vi "nanocal -- nuclear schottky fit V5.vi"() -> ()   [LabVIEW 2020] (continued)
                tunnel: [w595] -> w572 mode=indexing
                tunnel: w557 -> [w594] mode=indexing
                i -> [w596]
                n260 = Number To Fractional String(number=w594, precision (6)=i16 3) -> (F-format string=w595:string)  [unwired: 2 in]
                n261 = Insert Into Map(map in=w598, key=w596, value=w594) -> (map out=w597:map{i32, dbl})  [unwired: 2 out]
              }
              n262 = property on="θ (deg)" class="Ring (strict)"("Strings []"=w571) -> ()  [unwired: 2 in, 2 out]
              n263 = property on="B (T)" class="Ring (strict)"("Strings []"=w572) -> ()  [unwired: 2 in, 2 out]
              n264 = in-place-cluster #4("lookup.all set of"=w561, "lookup.all sides"=w560, "lookup.all T's"=w559, "lookup.all θ's"=w558, "lookup.all B's"=w557, "lookup.set of lookup"=w566, "lookup.side lookup"=w565, "lookup.T lookup"=w563, "lookup.B lookup"=w564, "lookup.θ lookup"=w562) -> (w541:T15)
            }
            n265 = for {
              tunnel: w545 -> [w609] mode=indexing
              shift-right: [w607] -> w543
              shift-left: w544 -> [w608]
              n266 = Unbundle(w609) -> ("event data"=w605:string, "file pattern"=w606:string)
              n267 = Insert Into Map(map in=w608, key=w606, value=w605) -> (map out=w607:map{string, string})  [unwired: 2 out]
            }
            n268 = local read "temps&degs"() -> (w549:map{string, map{T4, dbl}})
            n269 = local read "X selector"() -> (w548:T4)
            n270 = for {
              tunnel: [w618] -> w553 mode=indexing
              tunnel: [w622] -> w551 mode=indexing
              tunnel: [w619] -> w555 mode=indexing
              tunnel: w548 -> [w623]
              tunnel: w543 -> [w621] mode=indexing
              tunnel: w549 -> [w620]
              n271 = Unbundle(w621) -> (w618:string, w619:string)
              n272 = Look In Map(map=w620, key=w619) -> (value=w624:map{T4, dbl})  [unwired: 1 in, 1 out]
              n273 = Look In Map(map=w624, key=w623) -> (value=w622:dbl)  [unwired: 1 in, 1 out]
            }
            n274 = call "array - sorted inexes.vi"("x"=w551) -> ("index array"=w552:i32[])  [unwired: 9 in, 1 out]
            n275 = for {
              tunnel: w552 -> [w614] mode=indexing
              tunnel: w553 -> [w617]
              tunnel: [w616] -> w554 mode=indexing
              tunnel: w555 -> [w615]
              shift-right: [w610] -> w556
              shift-left: w550 -> [w613]
              i -> [w612]
              n276 = Index Array(array=w617, index=w614) -> (element=w616:string)
              n277 = Index Array(array=w615, index=w614) -> (element=w611:string)
              n278 = Insert Into Map(map in=w613, key=w612, value=w611) -> (map out=w610:map{i32, string})  [unwired: 2 out]
            }
            "filesnames lookup" <- w556
            n279 = property on="filenames" class="Ring (strict)"("Strings []"=w554) -> ()  [unwired: 2 in, 2 out]
            n280 = Generate User Event(user event=w546, event data cluster="action: update state of selectors" ("event data")) -> ()  [unwired: 2 in, 2 out]
            n281 = local write "selector"(w541) -> ()
          }
          frame "action: update constrained file selector" {
            w631 = map{i32, string} {}  # Size: 0
            n282 = local read "state of all selectors"() -> (w627:map{T4, map{bool, dbl}})
            n283 = local read "all short filenames"() -> (w628:map{string, string})
            n284 = local read "temps&degs"() -> (w629:map{string, map{T4, dbl}})
            n285 = for {
              tunnel: w628 -> [w641] mode=indexing
              tunnel: [w641] -> w630 mode=indexing if=w637
              shift-right: [w640] -> w626
              shift-left: w629 -> [w640]
              tunnel: w627 -> [w638]
              n286 = for {
                tunnel: [w653] -> w639 mode=indexing
                shift-right: [w648] -> _
                shift-left: w641 -> [w648]
                shift-right: [w647] -> _
                shift-left: w640 -> [w647]
                tunnel: w638 -> [w646] mode=indexing
                n287 = Unbundle(w648) -> ("event data"=w652:string)  [unwired: 1 out]
                n288 = Unbundle(w646) -> ("Plost: sweep window"=w645:T4, "map"=w644:map{bool, dbl})
                n289 = for {
                  tunnel: w644 -> [w656] mode=indexing
                  tunnel: [w655] -> w642
                  tunnel: [w654] -> w643
                  n290 = Unbundle(w656) -> ("ignore side !"=w655:bool, "number OUT"=w654:dbl)
                }
                n291 = Look In Map(map=w647, key=w652) -> (value=w651:map{T4, dbl})  [unwired: 1 in, 1 out]
                n292 = Look In Map(map=w651, key=w645) -> (value=w650:dbl)  [unwired: 1 in, 1 out]
                n293 = Equal?(x=w650, y=w643) -> (x = y?=w649:bool)
                n294 = Or(x=w642, y=w649) -> (x .or. y?=w653:bool)
              }
              n295 = And Array Elements(Boolean array=w639) -> (logical AND=w637:bool)
            }
            n296 = for {
              tunnel: [w671] -> w634 mode=indexing
              tunnel: [w669] -> w632 mode=indexing
              tunnel: [w666] -> w636 mode=indexing
              tunnel: w630 -> [w668] mode=indexing
              tunnel: w626 -> [w667]
              n297 = Unbundle(w668) -> ("event data"=w666:string, "file pattern"=w671:string)
              n298 = local read "X selector"() -> (w665:T4)
              n299 = Look In Map(map=w667, key=w666) -> (value=w670:map{T4, dbl})  [unwired: 1 in, 1 out]
              n300 = Look In Map(map=w670, key=w665) -> (value=w669:dbl)  [unwired: 1 in, 1 out]
            }
            n301 = call "array - sorted inexes.vi"("x"=w632) -> ("index array"=w633:i32[])  [unwired: 9 in, 1 out]
            n302 = for {
              tunnel: w633 -> [w661] mode=indexing
              tunnel: w634 -> [w664]
              tunnel: [w663] -> w635 mode=indexing
              tunnel: w636 -> [w662]
              shift-right: [w657] -> w625
              shift-left: w631 -> [w660]
              i -> [w659]
              n303 = Index Array(array=w664, index=w661) -> (element=w663:string)
              n304 = Index Array(array=w662, index=w661) -> (element=w658:string)
              n305 = Insert Into Map(map in=w660, key=w659, value=w658) -> (map out=w657:map{i32, string})  [unwired: 2 out]
            }
            "constrained filename lookup" <- w625
            n306 = property on="selection :|\\" class="Ring (strict)"("Strings []"=w635) -> ()  [unwired: 2 in, 2 out]
          }
          frame "action: constrained filenames select" {
            (unwired) 1
            n307 = local read "constrained filename lookup"() -> (w674:map{i32, string})
            n308 = local read "selection :|\\"() -> (w675:u16)
            n309 = local read "all full filenames"() -> (w676:map{string, path})
            n310 = Look In Map(map=w674, key=w675) -> (value=w677:string)  [unwired: 1 in, 1 out]
            n311 = Look In Map(map=w676, key=w677) -> (value=w678:path)  [unwired: 1 in, 1 out]
            n312 = local write "Read from file"(w678) -> ()
            n313 = Generate User Event(user event=w673, event data cluster="action: read from file" ("event data")) -> ()  [unwired: 2 in, 2 out]
          }
          frame "action: write mathematica string" {
            n314 = local read "mathematica thing"() -> (w683:map{string, map{T4, dbl}})
            n315 = local read "folder"() -> (w682:path)
            n316 = Build Path(base path=w682, name or relative path="temporarystring.txt") -> (appended path=w681:path)
            n317 = call "string parse mathematica list assosiated array -- V2.vi"("action"=3-lorentzian-heat-response_action."create string" ("derivative"), "Map IN"=w683) -> ("string out"=w679:string)  [unwired: 8 in, 1 out]
            "string OUT" <- w679
            n318 = Write to Text File(file (use dialog)=w681, text=w679) -> ()  [unwired: 2 in, 3 out]
          }
          frame "action: replot colors" {
            # "all -- including kappa0"
            n319 = local read "state of all selectors string"() -> (w692:string)
            n320 = local read "new selector names"() -> (w697:map{T4, map{T13, string}})
            n321 = local read "X selector"() -> (w693:T4)
            n322 = Look In Map(map=w697, key=w693) -> (value=w696:map{T13, string})  [unwired: 1 in, 1 out]
            n323 = local read "state of all selectors"() -> (w704:map{T4, map{bool, dbl}})
            n324 = local read "mathematica thing"() -> (w705:map{string, map{T4, dbl}})
            n325 = Look In Map(map=w696, key=nameformattingitem."nameL") -> (value=w694:string)  [unwired: 1 in, 1 out]
            n326 = Concatenate Strings(w692, w694) -> (w703:string)
            n327 = for {
              tunnel: w705 -> [w726]
              tunnel: w693 -> [w721]
              tunnel: w687 -> [w709] mode=indexing
              tunnel: w704 -> [w722]
              tunnel: w697 -> [w713]
              shift-right: [w717] -> w691
              shift-left: w703 -> [w720]
              tunnel: w692 -> [w718]
              tunnel: [w714] -> w690 mode=indexing
              n328 = for {
                tunnel: w726 -> [w740] mode=indexing
                tunnel: w709 -> [w739]
                tunnel: [w738] -> w725 mode=indexing if=w732
                tunnel: [w737] -> w724 mode=indexing if=w732
                tunnel: w721 -> [w736]
                tunnel: w722 -> [w735]
                n329 = Unbundle(w740) -> ("Map"=w734:map{T4, dbl})  [unwired: 1 out]
                n330 = for {
                  tunnel: w735 -> [w749] mode=indexing
                  tunnel: w734 -> [w748]
                  tunnel: [w746] -> w733 mode=indexing
                  n331 = Unbundle(w749) -> ("Plost: sweep window"=w747:T4, "map"=w745:map{bool, dbl})
                  n332 = for {
                    tunnel: w745 -> [w752] mode=indexing
                    tunnel: [w751] -> w742
                    tunnel: [w750] -> w743
                    n333 = Unbundle(w752) -> ("ignore side !"=w751:bool, "number OUT"=w750:dbl)
                  }
                  n334 = Look In Map(map=w748, key=w747) -> (value=w744:dbl)  [unwired: 1 in, 1 out]
                  n335 = Equal?(x=w744, y=w743) -> (x = y?=w741:bool)
                  n336 = Or(x=w742, y=w741) -> (x .or. y?=w746:bool)
                }
                n337 = Look In Map(map=w734, key=w736) -> (value=w738:dbl)  [unwired: 1 in, 1 out]
                n338 = Look In Map(map=w734, key=w739) -> (value=w737:dbl)  [unwired: 1 in, 1 out]
                n339 = And Array Elements(Boolean array=w733) -> (logical AND=w732:bool)
              }
              n340 = Look In Map(map=w713, key=w709) -> (value=w711:map{T13, string})  [unwired: 1 in, 1 out]
              n341 = Look In Map(map=w711, key=nameformattingitem."nameL") -> (value=w710:string)  [unwired: 1 in, 1 out]
              n342 = call <vilib>:"Space Constant.vi"() -> ("String"=w719:string)
              n343 = Concatenate Strings(w720, w719, w718, w710) -> (w717:string)
              n344 = call "array - sorted inexes.vi"("x"=w725) -> ("index array"=w723:i32[])  [unwired: 9 in, 1 out]
              n345 = for {
                tunnel: w725 -> [w731]
                tunnel: w724 -> [w730]
                tunnel: w723 -> [w727] mode=indexing
                tunnel: [w729] -> w716 mode=indexing
                tunnel: [w728] -> w715 mode=indexing
                n346 = Index Array(array=w731, index=w727) -> (element=w729:dbl)
                n347 = Index Array(array=w730, index=w727) -> (element=w728:dbl)
              }
              n348 = Bundle(w716, w715) -> (w714:cluster{dbl[], dbl[]})  [unwired: 1 in]
            }
            n349 = local read "folder"() -> (w702:path)
            n350 = Concatenate Strings("plotstring", w692, ".dat") -> (w698:string)
            n351 = Build Path(base path=w702, name or relative path=w698) -> (appended path=w701:path)
            n352 = call "nanocal -- plotstring file manage.vi"("Enum"=nanocal_--_plotstring_file_action."generate plotstring thing", "all data"=w690, "header line"=w691) -> ("plotstring thing"=w688:string)  [unwired: 8 in]
            n353 = flat-sequence {
              tunnel: w690 -> [w706]
              tunnel: w686 -> [w708]
              tunnel: "interface: replot colors plot" ("event data") -> [w707]
              frame #0 {
                "color data" <- w706
              }
              frame #1 {
                n354 = Generate User Event(user event=w708, event data cluster=w707) -> ()  [unwired: 2 in, 2 out]
              }
            }
            n355 = Write to Text File(file (use dialog)=w701, text=w688) -> ()  [unwired: 2 in, 3 out]
          }
          frame "action: update state of selectors" {
            w773 = T4[] [enum."T (K)", enum."B (T)", enum."θ (deg)", enum."side (S|R)"] items=["ζ", "τ1", "τS", "τN", "τC", "κ0", "m1", "m2", "m3", "T (K)", "B (T)", "θ (deg)", "side (S|R)", "set of (B|T)", "Re(offset)", "Im(offset)"]
            n356 = local read "selector"() -> (w769:T15)
            n357 = Unbundle By Name(w769) -> ("side (8S|4R)"=w768:i32, "ignore side !"=w767:bool, "lookup.side lookup"=w766:map{i32, dbl}, "T (K)"=w763:u16, "ignore T !"=w765:bool, "lookup.T lookup"=w764:map{i32, dbl}, "B (T)"=w760:u16, "ignore B !"=w762:bool, "lookup.B lookup"=w761:map{i32, dbl}, "θ (deg)"=w758:u16, "ignore θ !"=w757:bool, "lookup.θ lookup"=w759:map{i32, dbl}, "set (1T|2B)"=w754:i32, "ignore set of !"=w755:bool, "lookup.set of lookup"=w756:map{i32, dbl})
            n358 = Look In Map(map=w766, key=w768) -> (value=w772:dbl)  [unwired: 1 in, 1 out]
            n359 = local read "new selector names"() -> (w776:map{T4, map{T13, string}})
            n360 = node(w767, w772) -> (w793:map{bool, dbl})
            n361 = Look In Map(map=w764, key=w763) -> (value=w792:dbl)  [unwired: 1 in, 1 out]
            n362 = Look In Map(map=w761, key=w760) -> (value=w788:dbl)  [unwired: 1 in, 1 out]
            n363 = node(w765, w792) -> (w790:map{bool, dbl})
            n364 = node(w762, w788) -> (w787:map{bool, dbl})
            n365 = Look In Map(map=w759, key=w758) -> (value=w786:dbl)  [unwired: 1 in, 1 out]
            n366 = node(w757, w786) -> (w784:map{bool, dbl})
            n367 = Look In Map(map=w756, key=w754) -> (value=w783:dbl)  [unwired: 1 in, 1 out]
            n368 = local read "side map from NUM"() -> (w770:map{i32, T11})
            n369 = node(w755, w783) -> (w781:map{bool, dbl})
            n370 = node(3-lorentzian-parameters."side (S|R)" ("Plost: sweep window"), w793, 3-lorentzian-parameters."T (K)" ("Plost: sweep window"), w790, 3-lorentzian-parameters."B (T)" ("Plost: sweep window"), w787, 3-lorentzian-parameters."θ (deg)" ("Plost: sweep window"), w784, 3-lorentzian-parameters."set of (B|T)" ("Plost: sweep window"), w781) -> (w753:map{T4, map{bool, dbl}})
            "state of all selectors" <- w753
            n371 = for {
              tunnel: w776 -> [w798]
              shift-right: [w801] -> w774
              shift-left: "_" ("event data") -> [w800]
              tunnel: w773 -> [w797] mode=indexing
              tunnel: w753 -> [w795]
              n372 = Look In Map(map=w795, key=w797) -> (value=w803:map{bool, dbl})  [unwired: 1 in, 1 out]
              n373 = Look In Map(map=w798, key=w797) -> (value=w796:map{T13, string})  [unwired: 1 in, 1 out]
              n374 = for {
                tunnel: w803 -> [w818] mode=indexing
                tunnel: [w817] -> w802
                tunnel: [w816] -> w799
                n375 = Unbundle(w818) -> ("ignore side !"=w817:bool, "number OUT"=w816:dbl)
              }
              n376 = case shown="False" w802 {
                tunnel: [w814 w815] -> w801
                tunnel: w800 -> [w813 w815]
                tunnel: w799 -> [w810 _]
                tunnel: w796 -> [w806 _]
                frame False {
                  n377 = Look In Map(map=w806, key=nameformattingitem."units") -> (value=w807:string)  [unwired: 1 in, 1 out]
                  n378 = Look In Map(map=w806, key=nameformattingitem."prec") -> (value=w804:string)  [unwired: 1 in, 1 out]
                  n379 = Format Value(format string=w804, value (0)=w810) -> (output string=w809:string)  [unwired: 1 in]
                  n380 = Concatenate Strings(w813, "_" ("event data"), w809, w807, "_" ("event data")) -> (w814:string)
                }
                frame True {
                }
              }
            }
            "state of all selectors string" <- w774
            n381 = Look In Map(map=w770, key=w772) -> (value=w771:T11)  [unwired: 1 in, 1 out]
            n382 = local write "side"(w771) -> ()
            n383 = Generate User Event(user event=w777, event data cluster="action: replot colors" ("event data")) -> (user event out=w778:refnum<user-event>)  [unwired: 2 in, 1 out]
            n384 = Generate User Event(user event=w778, event data cluster="action: update constrained file selector" ("event data")) -> ()  [unwired: 2 in, 2 out]
          }
          frame "action: copy from math" {
            w828 = map{T4, bool} {}  # Size: 0
            n385 = local read "default selector"() -> (w827:T14)
            n386 = local read "mathematica thing"() -> (w833:map{string, map{T4, dbl}})
            n387 = case shown="True" "overwrite offset" {
              tunnel: w825 -> [w836 w840]
              tunnel: [w836 w839] -> w824
              frame False {
              }
              frame True {
                n388 = Build Array (concatenate)(w840, 3-lorentzian-parameters."Re(offset)" ("Plost: sweep window"), 3-lorentzian-parameters."Im(offset)" ("Plost: sweep window")) -> (w839:T4[])
              }
            }
            n389 = for {
              shift-right: [w844] -> w826
              shift-left: w828 -> [w845]
              tunnel: w827 -> [w843] mode=indexing
              n390 = Unbundle(w843) -> ("Plost: sweep window"=w842:T4, "used default"=w841:bool)
              n391 = Insert Into Map(map in=w845, key=w842, value=w841) -> (map out=w844:map{T4, bool})  [unwired: 2 out]
            }
            n392 = local read "key"() -> (w832:string)
            n393 = local read "parameter map"() -> (w821:map{T4, dbl})
            n394 = Look In Map(map=w833, key=w832) -> (key not found?=w830:bool, value=w831:map{T4, dbl})  [unwired: 1 in]
            n395 = case shown="False" w830 {
              tunnel: w831 -> [w859 _]
              tunnel: w826 -> [w857 _]
              tunnel: w824 -> [w858 _]
              tunnel: "overwrite offset" -> [w851 w894]
              tunnel: [w850 w894] -> w822
              tunnel: w821 -> [w849 _]
              tunnel: w819 -> [w847 _]
              frame False {
                # "the order of numbers \nMUST corrspond to order\nin the \"parameter\" array"
                n396 = for {
                  tunnel: [w869] -> w856 mode=indexing
                  tunnel: w859 -> [w877]
                  tunnel: w858 -> [w870] mode=indexing
                  tunnel: w857 -> [w876]
                  shift-right: [w871] -> w848
                  shift-left: w849 -> [w872]
                  n397 = Look In Map(map=w876, key=w870, default value=FALSE) -> (value=w875:bool)  [unwired: 1 out]
                  n398 = Look In Map(map=w877, key=w870) -> (value=w874:dbl)  [unwired: 1 in, 1 out]
                  n399 = case shown="True" w875 {
                    tunnel: w874 -> [w880 _]
                    tunnel: w870 -> [_ w881]
                    tunnel: [w880 w882] -> w869
                    frame False {
                    }
                    frame True {
                      n400 = local read "T (K)"() -> (w893:dbl)
                      n401 = local read "B (T)"() -> (w889:dbl)
                      n402 = Divide(x=w889, y=12.0) -> (x/y=w887:dbl)
                      n403 = Equal?(x=3-lorentzian-parameters."τN", y=w881) -> (x = y?=w890:bool)
                      n404 = Square(x=w887) -> (x^2=w886:dbl)
                      n405 = call "nanocal -- defaut parameter manager -- V1.vi"("action"=nanocal_--_defaut_parameter_manager_action--_V1."get logarithmic interp", "T"=w893, "what"=w881) -> ("number"=w884:dbl)  [unwired: 8 in]
                      n406 = Select(t=w886, s=w890, f=1.0) -> (s? t:f=w883:dbl)
                      n407 = Multiply(x=w884, y=w883) -> (x*y=w882:dbl)
                    }
                  }
                  n408 = in-place {
                    in-place-border: w869 -> [w879]
                    in-place-border: LVMapReplaceAction."Modify Entry only if found" ("action") -> [w878]
                    n409 = in-place-map #5(w872, w870) -> ()  [unwired: 1 in, 2 out]
                    n410 = in-place-map #5(w879, w878) -> (w871:map{T4, dbl})  [unwired: 2 out]
                  }
                }
                n411 = flat-sequence {
                  tunnel: w848 -> [w860]
                  tunnel: w847 -> [w862]
                  tunnel: "interface: update list from parameter map" ("event data") -> [w861]
                  frame #0 {
                    n412 = local write "parameter map"(w860) -> ()
                  }
                  frame #1 {
                    n413 = Generate User Event(user event=w862, event data cluster=w861) -> ()  [unwired: 2 in, 2 out]
                  }
                }
                n414 = Index Array(array=w856, index #1=6 ("index"), index #2=7 ("index")) -> (element #1=w853:dbl, element #2=w852:dbl)
                n415 = case shown="True" w851 {
                  selector: w851 -> [w863 w864]
                  tunnel: w853 -> [_ w866]
                  tunnel: w852 -> [_ w865]
                  tunnel: [w863 w864] -> w850
                  frame False {
                  }
                  frame True {
                    n416 = Bundle("number"=w866, "number"=w865) -> (w867:cluster{"number":dbl, "number":dbl})  [unwired: 1 in]
                    n417 = local write "offset Re\noffset Im"(w867) -> ()
                  }
                }
              }
              frame True {
              }
            }
            n418 = case shown="True" w822 {
              tunnel: ["action: new sweep" ("event data") "action: read from file" ("event data")] -> w820
              frame False {
              }
              frame True {
              }
            }
            n419 = Generate User Event(user event=w829, event data cluster=w820) -> ()  [unwired: 2 in, 2 out]
          }
          frame "action: copy to math" {
            w902 = T4[] [enum."T (K)", enum."B (T)", enum."θ (deg)", enum."Re(offset)", enum."Im(offset)"] items=["ζ", "τ1", "τS", "τN", "τC", "κ0", "m1", "m2", "m3", "T (K)", "B (T)", "θ (deg)", "side (S|R)", "set of (B|T)", "Re(offset)", "Im(offset)"]
            n420 = local read "offset Re\noffset Im"() -> (w898:cluster{"Numeric":dbl, "Numeric":dbl})
            n421 = local read "parameter map"() -> (w895:map{T4, dbl})
            n422 = local read "θ (deg)"() -> (w904:dbl)
            n423 = local read "T (K)"() -> (w906:dbl)
            n424 = local read "B (T)"() -> (w905:dbl)
            n425 = Unbundle(w898) -> ("Numeric"=w897:dbl, "Numeric"=w896:dbl)
            n426 = Build Array(w906, w905, w904, w897, w896) -> (w903:dbl[])
            n427 = for {
              tunnel: w903 -> [w912] mode=indexing
              tunnel: w902 -> [w913] mode=indexing
              shift-right: [w914] -> w901
              shift-left: w895 -> [w915]
              n428 = Insert Into Map(map in=w915, key=w913, value=w912) -> (map out=w914:map{T4, dbl})  [unwired: 2 out]
            }
            n429 = local read "mathematica thing"() -> (w909:map{string, map{T4, dbl}})
            n430 = local read "key"() -> (w908:string)
            n431 = call "3-lorentzian-heat-response -- V4.vi"("action"=3-lorentzian-heat-response_action."calc m1m2m3", "Map IN"=w901) -> ("Map OUT"=w900:map{T4, dbl})  [unwired: 7 in, 2 out]
            n432 = in-place {
              in-place-border: w900 -> [w916]
              n433 = in-place-map #6(w909, w908) -> (w919:map{T4, dbl})  [unwired: 1 in, 1 out]
              n434 = for {
                tunnel: w916 -> [w921] mode=indexing
                shift-right: [w924] -> w918
                shift-left: w919 -> [w925]
                shift-right: [w923] -> _
                shift-left: w916 -> [w923]
                n435 = Unbundle(w921) -> ("X selector"=w920:T4)  [unwired: 1 out]
                n436 = Look In Map(map=w923, key=w920) -> (value=w922:dbl)  [unwired: 1 in, 1 out]
                n437 = Insert Into Map(map in=w925, key=w920, value=w922) -> (map out=w924:map{T4, dbl})  [unwired: 2 out]
              }
              n438 = in-place-map #6(w918, LVMapReplaceAction."Modify Entry only if found" ("action")) -> (w907:map{string, map{T4, dbl}})  [unwired: 2 out]
            }
            n439 = local write "mathematica thing"(w907) -> ()
            n440 = Generate User Event(user event=w910, event data cluster="action: replot colors" ("event data")) -> ()  [unwired: 2 in, 2 out]
          }
          frame "action: exit" {
          }
          frame "action: read from file" {
            n441 = local read "Read from file"() -> (w927:path)
            n442 = local read "cursor x selector"() -> (w950:map{T4, dbl})
            n443 = call "file - read-write - list of lines-V2.vi"("read/write control"=file_--_read-write_control."read", "file path"=w927) -> ("header OUT"=w937:string, "list of lines OUT"=w939:string[], "filename out"=w967:string)  [unwired: 7 in]
            n444 = Unbundle("offset Re\noffset Im") -> ("Numeric"=w953:dbl, "Numeric"=w952:dbl)
            n445 = call "filename-manage.vi"("filename-action"=filename-action."get name", "file name IN"=w967) -> ("string OUT"=w936:string)  [unwired: 7 in, 2 out]
            n446 = Re/Im To Complex(1:w952, 2:w953) -> (0:w940:cdb)
            n447 = call "filename-manage.vi"("filename-action"=filename-action."get T", "file name IN"=w936) -> ("number OUT"=w949:dbl, "filename OUT"=w964:string)  [unwired: 7 in, 1 out]
            "T (K)" <- w949
            n448 = case shown="\"raw nanocal\"" "data file formatting" {
              tunnel: [w973 w991 w1027 w1054] -> w961
              tunnel: [w972 w990 w1026 w1053] -> w955
              tunnel: w940 -> [w971 w993 w1022 w1043]
              tunnel: w939 -> [w974 w1001 w1021 w1042]
              tunnel: w937 -> [_ w1002 _ _]
              tunnel: w936 -> [_ w989 _ _]
              tunnel: w927 -> [_ w992 _ _]
              tunnel: "side" -> [_ w988 _ _]
              tunnel: "toggle generate labview files" -> [_ w986 _ _]
              frame "as is", Default {
                n449 = for {
                  tunnel: w974 -> [w985] mode=indexing
                  tunnel: [w980] -> w975 mode=indexing if=w976
                  tunnel: [w979] -> w973 mode=indexing if=w976
                  w981 = 0.0
                  n450 = Scan From String(format string="%f%f%f", input string=w985, initial scan location=u32 0, default 1=w981, default 2=w981, default 3=w981) -> (offset past scan=w977:u32, output 1=w979:dbl, output 2=w983:dbl, output 3=w982:dbl)  [unwired: 1 in, 2 out]
                  n451 = Greater Than 0?(x=w977) -> (x > 0?=w976:bool)
                  n452 = Re/Im To Complex(1:w982, 2:w983) -> (0:w980:cdb)
                }
                n453 = Subtract(x=w975, y=w971) -> (x-y=w972:cdb[])
              }
              frame "raw nanocal" {
                n454 = case shown="\"ref\"" w988 {
                  tunnel: [nanocal_raw_file_manage_action_V1."read S side" ("action") nanocal_raw_file_manage_action_V1."read R side" ("action")] -> w987
                  frame "sam", Default {
                  }
                  frame "ref" {
                  }
                }
                n455 = call "nanocal_raw_file_manage_V1.vi"("action"=w987, "list of lines IN"=w1001, "header IN"=w1002) -> ("z (K/W)  OUT"=w994:cdb[], "f (Hz) OUT"=w995:dbl[])  [unwired: 6 in, 1 out]
                n456 = Subtract(x=w994, y=w993) -> (x-y=w996:cdb[])
                n457 = call "array -- freq-voltage transformations.vi"("freq voltage action"=array_--_freq-voltage_transformations_action."add -ω", "z In"=w996, "ω IN"=w995) -> ("z out"=w999:cdb[], "ω out"=w1000:dbl[])  [unwired: 5 in, 2 out]
                n458 = call "array -- freq-voltage transformations.vi"("freq voltage action"=array_--_freq-voltage_transformations_action."sort ω", "z In"=w999, "ω IN"=w1000) -> ("z out"=w990:cdb[], "ω out"=w991:dbl[])  [unwired: 5 in, 2 out]
                n459 = case shown="True" w986 {
                  tunnel: w992 -> [_ w1014]
                  tunnel: w989 -> [_ w1018]
                  tunnel: w991 -> [_ w1010]
                  tunnel: w990 -> [_ w1009]
                  frame False {
                  }
                  frame True {
                    n460 = call "filename-manage.vi"("filename-action"=filename-action."get basename", "file name IN"=w1018) -> ("string OUT"=w1016:string)  [unwired: 7 in, 2 out]
                    n461 = Strip Path(path=w1014) -> (stripped path=w1013:path)  [unwired: 1 out]
                    n462 = Concatenate Strings(w1016, "_labview_.dat") -> (w1005:string)
                    n463 = call "array -- freq-voltage transformations.vi"("freq voltage action"=array_--_freq-voltage_transformations_action."labview file str", "z In"=w1009, "ω IN"=w1010) -> ("lines out"=w1007:string[], "header OUT"=w1008:string)  [unwired: 5 in, 2 out]
                    n464 = Build Path(base path=w1013, name or relative path=w1005) -> (appended path=w1012:path)
                    n465 = call "file - read-write - list of lines-V2.vi"("read/write control"=file_--_read-write_control."write all", "header IN"=w1008, "list of lines IN"=w1007, "file path"=w1012) -> ()  [unwired: 5 in, 3 out]
                  }
                }
              }
              frame "add - ω" {
                n466 = for {
                  tunnel: w1021 -> [w1039] mode=indexing
                  tunnel: [w1034] -> w1023 mode=indexing if=w1030
                  tunnel: [w1033] -> w1019 mode=indexing if=w1030
                  w1035 = 0.0
                  n467 = Scan From String(format string="%f%f%f", input string=w1039, initial scan location=u32 0, default 1=w1035, default 2=w1035, default 3=w1035) -> (offset past scan=w1031:u32, output 1=w1033:dbl, output 2=w1037:dbl, output 3=w1036:dbl)  [unwired: 1 in, 2 out]
                  n468 = Greater Than 0?(x=w1031) -> (x > 0?=w1030:bool)
                  n469 = Re/Im To Complex(1:w1036, 2:w1037) -> (0:w1034:cdb)
                }
                n470 = Subtract(x=w1023, y=w1022) -> (x-y=w1020:cdb[])
                n471 = call "array -- freq-voltage transformations.vi"("freq voltage action"=array_--_freq-voltage_transformations_action."add -ω", "z In"=w1020, "ω IN"=w1019) -> ("z out"=w1028:cdb[], "ω out"=w1029:dbl[])  [unwired: 5 in, 2 out]
                n472 = call "array -- freq-voltage transformations.vi"("freq voltage action"=array_--_freq-voltage_transformations_action."sort ω", "z In"=w1028, "ω IN"=w1029) -> ("z out"=w1026:cdb[], "ω out"=w1027:dbl[])  [unwired: 5 in, 2 out]
              }
              frame "full rydh" {
                n473 = for {
                  tunnel: w1042 -> [w1066] mode=indexing
                  tunnel: [w1061] -> w1044 mode=indexing if=w1057
                  tunnel: [w1060] -> w1040 mode=indexing if=w1057
                  w1062 = 0.0
                  n474 = Scan From String(format string="%f%f%f", input string=w1066, initial scan location=u32 0, default 1=w1062, default 2=w1062, default 3=w1062) -> (offset past scan=w1058:u32, output 1=w1060:dbl, output 2=w1064:dbl, output 3=w1063:dbl)  [unwired: 1 in, 2 out]
                  n475 = Greater Than 0?(x=w1058) -> (x > 0?=w1057:bool)
                  n476 = Re/Im To Complex(1:w1063, 2:w1064) -> (0:w1061:cdb)
                }
                n477 = Subtract(x=w1044, y=w1043) -> (x-y=w1041:cdb[])
                n478 = call "array -- freq-voltage transformations.vi"("freq voltage action"=array_--_freq-voltage_transformations_action."2 x ω", "z In"=w1041, "ω IN"=w1040) -> ("z out"=w1048:cdb[], "ω out"=w1050:dbl[])  [unwired: 5 in, 2 out]
                n479 = call "array -- freq-voltage transformations.vi"("freq voltage action"=array_--_freq-voltage_transformations_action."R-phase(deg) to Re-Im", "z In"=w1048, "ω IN"=w1050) -> ("z out"=w1047:cdb[], "ω out"=w1049:dbl[])  [unwired: 5 in, 2 out]
                n480 = call "array -- freq-voltage transformations.vi"("freq voltage action"=array_--_freq-voltage_transformations_action."add -ω", "z In"=w1047, "ω IN"=w1049) -> ("z out"=w1055:cdb[], "ω out"=w1056:dbl[])  [unwired: 5 in, 2 out]
                n481 = call "array -- freq-voltage transformations.vi"("freq voltage action"=array_--_freq-voltage_transformations_action."sort ω", "z In"=w1055, "ω IN"=w1056) -> ("z out"=w1053:cdb[], "ω out"=w1054:dbl[])  [unwired: 5 in, 2 out]
              }
            }
            n482 = Insert Into Map(map in=w950, key=3-lorentzian-parameters."T (K)" ("Plost: sweep window"), value=w949) -> (map out=w948:map{T4, dbl})  [unwired: 2 out]
            n483 = call "filename-manage.vi"("filename-action"=filename-action."get deg", "file name IN"=w964) -> ("number OUT"=w945:dbl, "filename OUT"=w931:string)  [unwired: 7 in, 1 out]
            "θ (deg)" <- w945
            n484 = local read "side map to STR"() -> (w929:map{T11, string})
            n485 = Insert Into Map(map in=w948, key=3-lorentzian-parameters."θ (deg)" ("Plost: sweep window"), value=w945) -> (map out=w947:map{T4, dbl})  [unwired: 2 out]
            n486 = call "filename-manage.vi"("filename-action"=filename-action."get B", "file name IN"=w931) -> ("number OUT"=w944:dbl, "filename OUT"=w930:string)  [unwired: 7 in, 1 out]
            "B (T)" <- w944
            n487 = call "filename-manage.vi"("filename-action"=filename-action."getIDStock", "file name IN"=w930) -> ("string OUT"=w934:string)  [unwired: 7 in, 2 out]
            "file IDS" <- w934
            n488 = Look In Map(map=w929, key="side") -> (value=w935:string)  [unwired: 1 in, 1 out]
            n489 = Insert Into Map(map in=w947, key=3-lorentzian-parameters."B (T)" ("Plost: sweep window"), value=w944) -> (map out=w946:map{T4, dbl})  [unwired: 2 out]
            n490 = Concatenate Strings(w934, w935) -> (→"key":string)
            n491 = local write "cursor x selector"(w946) -> ()
            n492 = call "filter - complex - four.vi"("omega (Hz) in"=w961, "z in"=w955, "span"="cspan") -> ("omega out"=w960:dbl[], "z out"=w959:cdb[], "dz/domega out"=w958:cdb[])  [unwired: 9 in, 5 out]
            n493 = call "nanocal -- publish -- freq scan V2.vi"("publisher action"=publisher_action."set", "dz/dω IN (V)"=w958, "z IN (V)"=w959, "ω IN (Hz)"=w960) -> ()  [unwired: 4 in, 4 out]
            n494 = Generate User Event(user event=w968, event data cluster="action: new sweep" ("event data")) -> ()  [unwired: 2 in, 2 out]
          }
          frame "action: save freq scan" {
            n495 = local read "Freq sweep name template"() -> (w1072:T10)
            n496 = call "MFLI -- publish -- freq scan.vi"("publisher action"=publisher_action."get") -> ("Voltage out (V)"=w1068:cdb[], "Freq out (Hz)"=w1069:dbl[])  [unwired: 9 in]
            n497 = call "filename-manage.vi"("filename pattern"=w1072, "filename-action"=filename-action."uniquenum", "folder IN"="Save folder", "file name IN"="freq sweep file name") -> ("filename OUT"=w1071:string)  [unwired: 5 in, 2 out]
            n498 = call "KM_appendline -- freq sweep.vi"("freq"=w1069, "Vout(V)"=w1068, "Save frequency scan"="Save folder", "read/write control"=KM_file_--_read-write_control."append one line", "name or relative path"=w1071) -> ()  [unwired: 15 in]
            n499 = local write "freq sweep file name"(w1071) -> ()
          }
          frame "void", Default {
          }
        }
      }
    }
  }
  n500 = while "interface actions" {
    tunnel: w9 -> [w1079]
    tunnel: w6 -> [w1077]
    tunnel: w5 -> [w1076]
    stop <- FALSE stop-if-true
    n501 = event shown="[1] <interface>: User Event" {
      selector: w1079 -> [_ _]
      dyn-events: _ -> [_ _]
      timeout: _ -> [_ _]
      tunnel: w1077 -> [_ w1081]
      tunnel: w1076 -> [_ w1080]
      event Timeout {
        n502 = event-data() -> ()  [unwired: 1 in, 3 out]
      }
      event User Event {
        n503 = event-data() -> ("interface"=w1082:string)  [unwired: 1 in]
        n504 = case shown="\"interface: update curvature plot\"" w1082 {
          tunnel: [_ _ _ _ _ _ _ _ _ _ TRUE] -> _
          tunnel: w1081 -> [_ _ w1103 w1135 _ _ w1204 w1235 _ _ _]
          tunnel: w1080 -> [_ _ _ _ w1153 _ _ _ _ _ _]
          frame "void", Default {
          }
          frame "interface: reset colors" {
            w1089 = map{T4, u32} {}  # Size: 0
            n505 = local read "parameter"() -> (w1092:T4[])
            n506 = local read "colors"() -> (w1090:u32[])
            n507 = for {
              shift-right: [w1101] -> w1091
              shift-left: w1089 -> [w1102]
              tunnel: w1092 -> [w1100] mode=indexing
              tunnel: w1090 -> [w1099] mode=indexing
              n508 = Insert Into Map(map in=w1102, key=w1100, value=w1099) -> (map out=w1101:map{T4, u32})  [unwired: 2 out]
            }
            n509 = local write "color Map"(w1091) -> ()
            n510 = Look In Map(map=w1091, key=3-lorentzian-parameters."ζ" ("Plost: sweep window")) -> (value=w1093:u32)  [unwired: 1 in, 1 out]
            n511 = Look In Map(map=w1091, key=3-lorentzian-parameters."τ1" ("Plost: sweep window")) -> (value=w1094:u32)  [unwired: 1 in, 1 out]
            n512 = Look In Map(map=w1091, key=3-lorentzian-parameters."τS" ("Plost: sweep window")) -> (value=w1095:u32)  [unwired: 1 in, 1 out]
            n513 = Look In Map(map=w1091, key=3-lorentzian-parameters."τN" ("Plost: sweep window")) -> (value=w1096:u32)  [unwired: 1 in, 1 out]
            n514 = Look In Map(map=w1091, key=3-lorentzian-parameters."τC" ("Plost: sweep window")) -> (value=w1097:u32)  [unwired: 1 in, 1 out]
            n515 = Look In Map(map=w1091, key=3-lorentzian-parameters."κ0" ("Plost: sweep window")) -> (value=w1098:u32)  [unwired: 1 in, 1 out]
            n516 = property on="ζ" class="Slide (strict)"("Fill Color"=w1093) -> ()  [unwired: 2 in, 2 out]
            n517 = property on="T1" class="Slide (strict)"("Fill Color"=w1094) -> ()  [unwired: 2 in, 2 out]
            n518 = property on="τS" class="Slide (strict)"("Fill Color"=w1095) -> ()  [unwired: 2 in, 2 out]
            n519 = property on="τN" class="Slide (strict)"("Fill Color"=w1096) -> ()  [unwired: 2 in, 2 out]
            n520 = property on="τC" class="Slide (strict)"("Fill Color"=w1097) -> ()  [unwired: 2 in, 2 out]
            n521 = property on="κ0" class="Slide (strict)"("Fill Color"=w1098) -> ()  [unwired: 2 in, 2 out]
          }
          frame "interface: update plot colors cursors" {
            w1108 = T4[] [enum."m1", enum."m2", enum."m3"] items=["ζ", "τ1", "τS", "τN", "τC", "κ0", "m1", "m2", "m3", "T (K)", "B (T)", "θ (deg)", "side (S|R)", "set of (B|T)", "Re(offset)", "Im(offset)"]
            w1106 = T4[] [enum."T (K)", enum."B (T)", enum."θ (deg)"] items=["ζ", "τ1", "τS", "τN", "τC", "κ0", "m1", "m2", "m3", "T (K)", "B (T)", "θ (deg)", "side (S|R)", "set of (B|T)", "Re(offset)", "Im(offset)"]
            n522 = local read "parameter map"() -> (w1121:map{T4, dbl})
            n523 = local read "cursor x selector"() -> (w1109:map{T4, dbl})
            n524 = local read "X selector"() -> (w1110:T4)
            n525 = local read "T (K)"() -> (w1111:dbl)
            n526 = local read "θ (deg)"() -> (w1116:dbl)
            n527 = local read "B (T)"() -> (w1115:dbl)
            n528 = local read "T (K)"() -> (w1114:dbl)
            n529 = call "3-lorentzian-heat-response -- V4.vi"("action"=3-lorentzian-heat-response_action."calc m1m2m3", "Map IN"=w1121) -> ("Map OUT"=w1117:map{T4, dbl})  [unwired: 7 in, 2 out]
            n530 = local read "parameter"() -> (w1122:T4[])
            n531 = local read "cursor index map"() -> (w1113:map{T4, i32})
            n532 = Look In Map(map=w1109, key=w1110, default value=w1111) -> (value=w1112:dbl)  [unwired: 1 out]
            n533 = Build Array(w1114, w1115, w1116) -> (w1104:dbl[])
            n534 = Build Array (concatenate)(w1122, w1108) -> (w1120:T4[])
            n535 = for {
              shift-right: [w1125] -> w1118
              shift-left: w1117 -> [w1126]
              tunnel: w1106 -> [w1124] mode=indexing
              tunnel: w1104 -> [w1123] mode=indexing
              n536 = Insert Into Map(map in=w1126, key=w1124, value=w1123) -> (map out=w1125:map{T4, dbl})  [unwired: 2 out]
            }
            n537 = for {
              tunnel: w1112 -> [w1134]
              tunnel: w1103 -> [w1133]
              tunnel: w1120 -> [w1129] mode=indexing
              tunnel: w1113 -> [w1131]
              shift-right: [w1128] -> _
              shift-left: w1117 -> [w1128]
              n538 = Look In Map(map=w1128, key=w1129) -> (value=w1127:dbl)  [unwired: 1 in, 1 out]
              n539 = Look In Map(map=w1131, key=w1129) -> (value=w1130:i32)  [unwired: 1 in, 1 out]
              n540 = call "replace cursor - plot ref - V2.vi"("Plot ref in"=w1133, "new X"=w1134, "new  Y"=w1127, "cursor index"=w1130, "cursor action"=cursor_action."write") -> ()  [unwired: 11 in, 4 out]
            }
            n541 = call "string parse mathematica assosiated array.vi"("action"=mathematica_string_map_action."create string" ("derivative"), "map IN"=w1118) -> ("String OUT"=w1119:string)  [unwired: 8 in, 1 out]
            n542 = local write "String"(w1119) -> ()
          }
          frame "interface: plot colors update m1m2m3 cursors" {
            w1136 = T4[] [enum."m1", enum."m2", enum."m3"] items=["ζ", "τ1", "τS", "τN", "τC", "κ0", "m1", "m2", "m3", "T (K)", "B (T)", "θ (deg)", "side (S|R)", "set of (B|T)", "Re(offset)", "Im(offset)"]
            n543 = local read "parameter map"() -> (w1144:map{T4, dbl})
            n544 = call "3-lorentzian-heat-response -- V4.vi"("action"=3-lorentzian-heat-response_action."calc m1m2m3", "Map IN"=w1144) -> ("Map OUT"=w1143:map{T4, dbl})  [unwired: 7 in, 2 out]
            n545 = local read "cursor x selector"() -> (w1138:map{T4, dbl})
            n546 = local read "X selector"() -> (w1139:T4)
            n547 = local read "cursor index map"() -> (w1142:map{T4, i32})
            n548 = local read "T (K)"() -> (w1140:dbl)
            n549 = Look In Map(map=w1138, key=w1139, default value=w1140) -> (value=w1141:dbl)  [unwired: 1 out]
            n550 = for {
              tunnel: w1141 -> [w1152]
              tunnel: w1136 -> [w1148] mode=indexing
              tunnel: w1142 -> [w1150]
              shift-right: [w1147] -> _
              shift-left: w1143 -> [w1147]
              tunnel: w1135 -> [w1145]
              n551 = Look In Map(map=w1147, key=w1148) -> (value=w1146:dbl)  [unwired: 1 in, 1 out]
              n552 = Look In Map(map=w1150, key=w1148) -> (value=w1149:i32)  [unwired: 1 in, 1 out]
              n553 = call "replace cursor - plot ref - V2.vi"("Plot ref in"=w1145, "new X"=w1152, "new  Y"=w1146, "cursor index"=w1149, "cursor action"=cursor_action."write") -> ()  [unwired: 11 in, 4 out]
            }
          }
          frame "interface: update circle fit plot" {
            n554 = for {
              N: 1 -> [_]
              tunnel: w1153 -> [w1155]
              n555 = local read "current plot ind"() -> (w1157:i32)
              n556 = local read "factors"() -> (w1165:cluster{"scaling":dbl, "what":T4}[])
              n557 = local read "vector v=dlogG/dlogα of logarithmic derivatives"() -> (w1160:dbl[])
              n558 = for {
                shift-right: [w1179] -> w1159
                shift-left: _ -> [w1180]
                tunnel: w1165 -> [w1178] mode=indexing
                n559 = Unbundle(w1178) -> ("scaling"=w1176:dbl, "what"=w1177:T4)
                n560 = Insert Into Map(map in=w1180, key=w1177, value=w1176) -> (map out=w1179:map{T4, dbl})  [unwired: 2 out]
              }
              n561 = local read "parameter"() -> (w1161:T4[])
              n562 = Increment(x=w1157) -> (x+1=w1156:i32)
              n563 = local read "R(ω) fit out"() -> (w1170:cdb[])
              n564 = Square(x=w1160) -> (x^2=w1163:dbl[])
              n565 = local write "current plot ind"(w1156) -> ()
              n566 = for {
                tunnel: w1161 -> [w1175] mode=indexing
                shift-right: [w1174] -> _
                shift-left: w1159 -> [w1174]
                tunnel: w1163 -> [w1172] mode=indexing
                tunnel: [w1171] -> w1162 mode=indexing
                n567 = Look In Map(map=w1174, key=w1175) -> (value=w1173:dbl)  [unwired: 1 in, 1 out]
                n568 = Multiply(x=w1173, y=w1172) -> (x*y=w1171:dbl)
              }
              n569 = Complex To Re/Im(x + iy=w1170) -> (x=w1168:dbl[], y=w1169:dbl[])
              n570 = Add Array Elements(numeric array=w1162) -> (sum=w1164:dbl)
              n571 = call "replace plot - plot ref - V2.vi"("Plot ref in"=w1155, "Array X IN"=w1168, "Array Y IN"=w1169, "plot index"=enum16{"data R(ω)", "fit R(ω)"}."fit R(ω)" ("Plost: sweep window"), "cursor action"=cursor_action."write") -> ()  [unwired: 11 in, 4 out]
              n572 = Square Root(x=w1164) -> (sqrt(x)=w1158:dbl)
              n573 = local write "|dln G/dln α_i |"(w1158) -> ()
            }
          }
          frame "interface: update curvature plot" {
            n574 = call "nanocal manage curvature plot.vi"("aggregator action"=agregator_--_action."interpolate") -> ("arrays OUT"=w1189:T35)  [unwired: 7 in, 3 out]
            n575 = control-ref of="Plot: curvature"() -> (w1182:refnum<vi>)
            n576 = Unbundle(w1189) -> ("Array"=w1188:dbl[], "Array"=w1187:dbl[])  [unwired: 1 out]
            n577 = Power Of 10(x=w1188) -> (10^x=w1184:dbl[])
            n578 = Power Of 10(x=w1187) -> (10^x=w1183:dbl[])
            n579 = call "replace plot - plot ref - V2.vi"("Plot ref in"=w1182, "Array X IN"=w1184, "Array Y IN"=w1183, "plot index"=0, "cursor action"=cursor_action."write") -> ()  [unwired: 11 in, 4 out]
            n580 = case shown="True" "update curvature plots" {
              tunnel: w1182 -> [_ w1201]
              frame False {
              }
              frame True {
                n581 = local read "newton parameters"() -> (w1199:T5)
                n582 = local read "parameter map"() -> (w1200:map{T4, dbl})
                n583 = call "nanocal -- publish -- freq scan V2.vi"("publisher action"=publisher_action."get") -> ("data"=w1192:T32)  [unwired: 7 in, 3 out]
                n584 = call "nanocal generate curvature ellipse.vi"("ellipse factor"="ellipse factor", "radius factor"="radius factor", "number of points"=20, "data"=w1192, "newton parameters"=w1199, "parameter map"=w1200) -> ("y OUT"=w1197:dbl[], "x OUT"=w1198:dbl[], "curvature tensor"=→"curvature tensor":T3)  [unwired: 3 in]
                n585 = call "replace plot - plot ref - V2.vi"("Plot ref in"=w1201, "Array X IN"=w1198, "Array Y IN"=w1197, "plot index"=1, "cursor action"=cursor_action."write") -> ()  [unwired: 11 in, 4 out]
              }
            }
          }
          frame "interface: replot colors plot" {
            n586 = local read "X selector"() -> (w1205:T4)
            n587 = local read "cursor index map"() -> (w1206:map{T4, i32})
            n588 = case shown="\"B (T)\"" w1205 {
              tunnel: ["B (T)" "T (K)"] -> w1211
              frame "B (T)" {
              }
              frame "T (K)", Default {
              }
            }
            n589 = local read "parameter"() -> (w1212:T4[])
            n590 = local read "color Map"() -> (w1207:map{T4, u32})
            n591 = local read "color data"() -> (w1208:cluster{"Array":dbl[], "Array":dbl[]}[])
            n592 = call "replace plot - plot ref - V2.vi"("Plot ref in"=w1204, "text"=w1211, "cursor action"=cursor_action."set Xlabel") -> ("Plot ref out"=w1209:refnum<vi>)  [unwired: 13 in, 3 out]
            n593 = for {
              tunnel: w1212 -> [w1221] mode=indexing
              tunnel: w1209 -> [w1220]
              tunnel: w1208 -> [w1219] mode=indexing
              tunnel: w1207 -> [w1216]
              tunnel: w1206 -> [w1215]
              n594 = Unbundle(w1219) -> ("Array"=w1217:dbl[], "Array"=w1218:dbl[])
              n595 = case shown="\"ζ\"..\"τC\", Default" w1221 {
                selector: w1221 -> [_ w1230]
                tunnel: w1217 -> [_ w1232]
                tunnel: w1218 -> [_ w1231]
                tunnel: w1216 -> [_ w1229]
                tunnel: w1215 -> [_ w1228]
                tunnel: w1220 -> [_ w1222]
                frame "κ0" {
                }
                frame "ζ".."τC", Default {
                  n596 = Look In Map(map=w1228, key=w1230) -> (value=w1224:i32)  [unwired: 1 in, 1 out]
                  n597 = call "replace plot - plot ref - V2.vi"("Plot ref in"=w1222, "Array X IN"=w1232, "Array Y IN"=w1231, "plot index"=w1224, "cursor action"=cursor_action."write") -> ("Plot ref out"=w1227:refnum<vi>)  [unwired: 11 in, 3 out]
                  n598 = Look In Map(map=w1229, key=w1230) -> (value=w1223:u32)  [unwired: 1 in, 1 out]
                  n599 = call "replace cursor - plot ref - V2.vi"("Plot ref in"=w1227, "cursor index"=w1224, "cursor action"=cursor_action."set cursor color", "Color Box"=w1223) -> ("Plot ref out"=w1226:refnum<vi>)  [unwired: 12 in, 3 out]
                  n600 = call "replace plot - plot ref - V2.vi"("Plot ref in"=w1226, "plot index"=w1224, "cursor action"=cursor_action."set plot color", "Color Box"=w1223) -> ()  [unwired: 12 in, 4 out]
                }
              }
            }
          }
          frame "interface: update color cursors" {
            w1237 = T4[] [enum."ζ", enum."τ1", enum."τS", enum."τN", enum."τC", enum."κ0", enum."m1", enum."m2", enum."m3"] items=["ζ", "τ1", "τS", "τN", "τC", "κ0", "m1", "m2", "m3", "T (K)", "B (T)", "θ (deg)", "side (S|R)", "set of (B|T)", "Re(offset)", "Im(offset)"]
            n601 = local read "parameter map"() -> (w1236:map{T4, dbl})
            n602 = local read "cursor x selector"() -> (w1239:map{T4, dbl})
            n603 = local read "X selector"() -> (w1240:T4)
            n604 = local read "T (K)"() -> (w1241:dbl)
            n605 = Look In Map(map=w1239, key=w1240, default value=w1241) -> (value=w1242:dbl)  [unwired: 1 out]
            n606 = local read "cursor index map"() -> (w1243:map{T4, i32})
            n607 = call "3-lorentzian-heat-response -- V4.vi"("action"=3-lorentzian-heat-response_action."calc m1m2m3", "Map IN"=w1236) -> ("Map OUT"=w1244:map{T4, dbl})  [unwired: 7 in, 2 out]
            n608 = for {
              tunnel: w1242 -> [w1252]
              tunnel: w1235 -> [w1251]
              tunnel: w1237 -> [w1247] mode=indexing
              tunnel: w1243 -> [w1249]
              shift-right: [w1246] -> _
              shift-left: w1244 -> [w1246]
              n609 = Look In Map(map=w1246, key=w1247) -> (value=w1245:dbl)  [unwired: 1 in, 1 out]
              n610 = Look In Map(map=w1249, key=w1247) -> (value=w1248:i32)  [unwired: 1 in, 1 out]
              n611 = call "replace cursor - plot ref - V2.vi"("Plot ref in"=w1251, "new X"=w1252, "new  Y"=w1245, "cursor index"=w1248, "cursor action"=cursor_action."write") -> ()  [unwired: 11 in, 4 out]
            }
          }
          frame "interface: update fit string" {
            w1255 = T4[] [enum."T (K)", enum."B (T)", enum."θ (deg)"] items=["ζ", "τ1", "τS", "τN", "τC", "κ0", "m1", "m2", "m3", "T (K)", "B (T)", "θ (deg)", "side (S|R)", "set of (B|T)", "Re(offset)", "Im(offset)"]
            n612 = local read "parameter map"() -> (w1253:map{T4, dbl})
            n613 = local read "θ (deg)"() -> (w1259:dbl)
            n614 = local read "B (T)"() -> (w1258:dbl)
            n615 = local read "T (K)"() -> (w1257:dbl)
